vi "Sort Packets.vi"(11 "Packets":string[](array[string])) -> (3 "Sorted Packets":string[](array[string]))   [LabVIEW 2021, in "d13.lvlib"]
uses:
  d13.lvlib
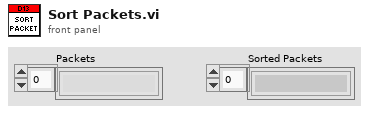
[diagram p1: front panel]
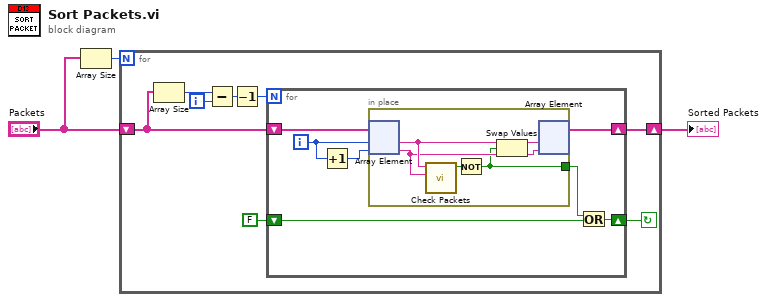
[diagram p0: block diagram]
diagram:
  n1 = Array Size(array="Packets") -> (size(s)=w1:i32)
  n2 = for {
    N: w1 -> [_]
    shift-right: [w8] -> w2
    shift-left: "Packets" -> [w11]
    i -> [w6]
    stop <- w4 continue-if-true
    n3 = Array Size(array=w11) -> (size(s)=w10:i32)
    n4 = Subtract(x=w10, y=w6) -> (x-y=w7:i32)
    n5 = Decrement(x=w7) -> (x-1=w9:i32)
    n6 = for {
      N: w9 -> [_]
      shift-right: [w17] -> w8
      shift-left: w11 -> [w18]
      shift-right: [w12] -> w4
      shift-left: FALSE -> [w14]
      i -> [w15]
      n7 = Increment(x=w15) -> (x+1=w16:i32)
      n8 = in-place {
        in-place-border: [w19] -> w13
        n9 = in-place-array #1(w18, w15, w16) -> (w24:string, w23:string)
        n10 = call "Check Packets.vi"("Right Packet"=w23, "Left Packet"=w24) -> ("Correct Order?"=w20:bool)  [unwired: 8 in, 1 out]
        n11 = Not(x=w20) -> (.not. x?=w19:bool)
        n12 = Swap Values(12:w24, 13:w19, 14:w23) -> (1:w22:string, 3:w21:string)
        n13 = in-place-array #1(w22, w21) -> (w17:string[])  [unwired: 2 out]
      }
      n14 = Or(x=w13, y=w14) -> (x .or. y?=w12:bool)
    }
  }
  "Sorted Packets" <- w2
